vi "tb_log 64bit number.vi"() -> ()   [LabVIEW 2011]
panel:
  out "Log Number":fxp<+/-,16,9>[](array[numeric])=[0.0, 0.0, 0.0, 0.0, 0.0, -189.6484375, -128.0, -128.0, -128.0, -128.0, -128.0, -128.0, -128.0, -128.0, -128.0, -189.6484375, -189.6484375, -189.6484375, -189.6484375, -189.6484375] format="%.10g"
  out "Mantissa (M)":fxp<+,64,0>=0.5 format="%.64g"
  out "Exponent (-N)":u8=62
  out "Output Valid":bool[](array[boolean])=[FALSE, FALSE, FALSE, FALSE, FALSE, FALSE, FALSE, FALSE, FALSE, FALSE, FALSE, FALSE, FALSE, FALSE, FALSE, TRUE, TRUE, TRUE, TRUE, TRUE]
  in  "Input Number (0.64)":fxp<+,64,0>=1.0842021724855044e-19 format="%.0b"
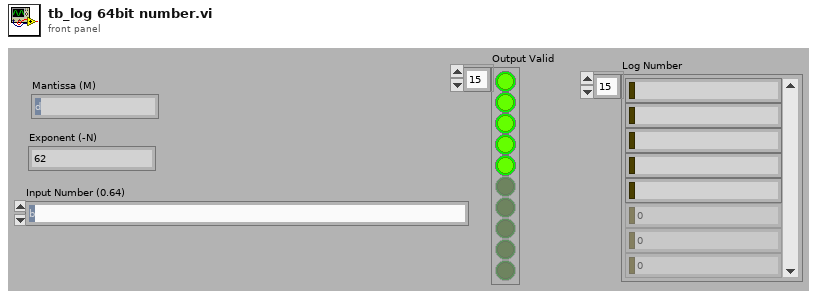
[diagram p1: front panel]
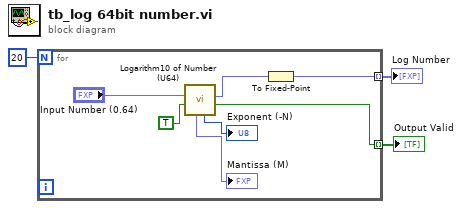
[diagram p0: block diagram]
diagram:
  n1 = for {
    N: 20 -> [_]
    tunnel: [w9] -> w2 mode=indexing
    tunnel: [w4] -> w1 mode=indexing
    n2 = call <userlib>:"Logarithm10 of Number (U64).vi"("Input Valid"=TRUE, "Input Number (0.64)"="Input Number (0.64)") -> ("Output Valid"=w9:bool, "Logarithm"=w5:fxp<+/-,34,12>, "Exponent (-N)"=→"Exponent (-N)":u8, "Mantissa (M)"=→"Mantissa (M)":fxp<+,64,0>)  [unwired: 6 in]
    n3 = To Fixed-Point(number=w5) -> (fixed-point=w4:fxp<+/-,16,9>)  [unwired: 1 in]
  }
  "Output Valid" <- w2
  "Log Number" <- w1
